vi "Execute Function.vi"(8 "error in":errorcluster, 10 "modbus request":refnum<class "Modbus Data Unit.lvclass">, 11 "device data model in":refnum<class "Device Data Model.lvclass">) -> (0 "error out":errorcluster, 2 "modbus response":refnum<class "Modbus Data Unit.lvclass">, 3 "device data model out":refnum<class "Device Data Model.lvclass">)   [LabVIEW 2014, in "MyLib.lvlib" / "Device Data Model.lvclass"]
doc: "This function is responsible for deciding what code to execute when a specific function is called."
uses:
  Device Data Model.lvclass
  Modbus Data Unit/Modbus Data Unit.lvclass
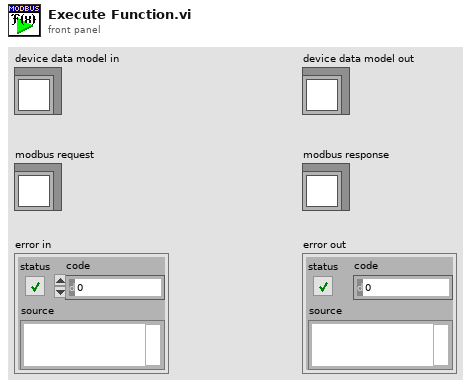
[diagram p1: front panel]
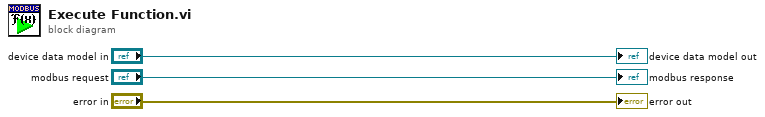
[diagram p0: block diagram]
diagram:
  "error out" <- "error in"
  "device data model out" <- "device data model in"
  "modbus response" <- "modbus request"
